vi "Add Scalar to Group.vi"(8 "error in":errorcluster, 10 "Scalar Data":T5, 11 "FPGA Addon refnum in":T2 format="%.0x") -> (0 "error out":errorcluster, 2 "Group Scalar Data out":T1 {"Scalar Section ref" format="%.0x"; "Group Section ref" format="%.0x"; "Group Scalar Registers"."Data Type" format="%.0x"}, 3 "FPGA Addon refnum out":T2=18446744073709551615 format="%.0x")   [LabVIEW 2019, in "Scripting API.lvlib"]
uses:
  Scripting API.lvlib
  TypeDefs/Input Scalar Data.ctl
  <vilib>/NI VeriStand/Custom Device API/Custom Device Item Ref.ctl
  TypeDefs/Group Scalar Data.ctl
  Addon/Addon Shared/Types/Register Information.ctl
  Addon/Addon Shared/Types/FPGA Addon Data Type.ctl
  Addon/Addon System Explorer/FPGA Addon System Explorer.lvlib
  Addon/Addon Shared/FPGA Addon Shared.lvlib
  <vilib>/NI VeriStand/Custom Device API/Custom Device API.lvlib
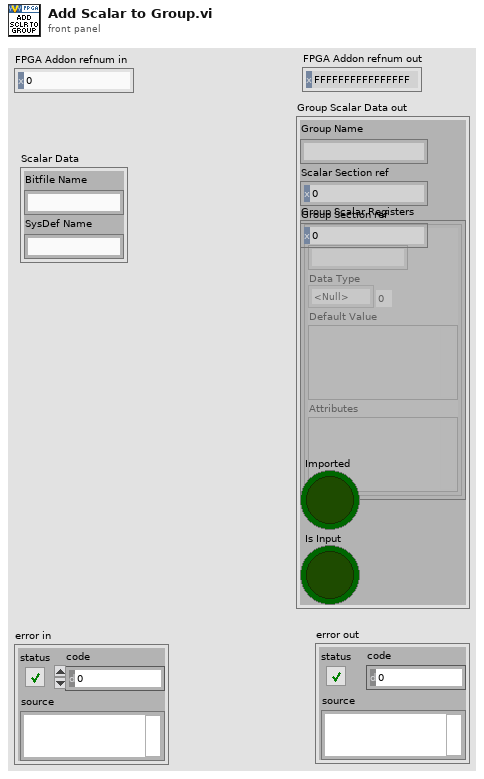
[diagram p1: front panel]
types:
  T1 = typedef "Scripting API.lvlib/Group Scalar Data.ctl" = cluster{"Group Name":string, "Scalar Section ref":T2, "Group Section ref":T2, "Group Scalar Registers":T3[], "Imported":bool, "Is Input":bool}
  T2 = typedef "Custom Device API.lvlib/Custom Device Item Ref.ctl" = u64
  T3 = typedef "FPGA Addon Shared.lvlib/Register Information.ctl" = cluster{"Name":string, "Data Type":T4, "Default Value":variant, "Attributes":variant}
  T4 = typedef "FPGA Addon Shared.lvlib/FPGA Addon Data Type.ctl" = enum8{"<Null>", "I8", "I16", "I32", "I64", "U8", "U16", "U32", "U64", "SGL", "Boolean", "Analog PWM In Settings", "Analog PWM In", "Digital PWM In Settings", "Digital PWM In", "Digital PWM Out", "Sine Out", "FXP", "FXP+/-24.5", "FXP+/-16.5", "FXP+/-32.8", "FXP+/-64.32", "FXP+/-16.7", "FXP+/-20.5", "FXP+/-27.5", "FXP+/-32.16", "FXP+16.3", "FXP+18.3", "Digital Static In", "Digital Static Out", "Digital Static In Settings", "Digital WSS Out", "Quad Encoder Settings", "Quad Encoder In", "Group"}
  T5 = typedef "Scripting API.lvlib/Input Scalar Data.ctl" = cluster{"Bitfile Name":string, "SysDef Name":string}
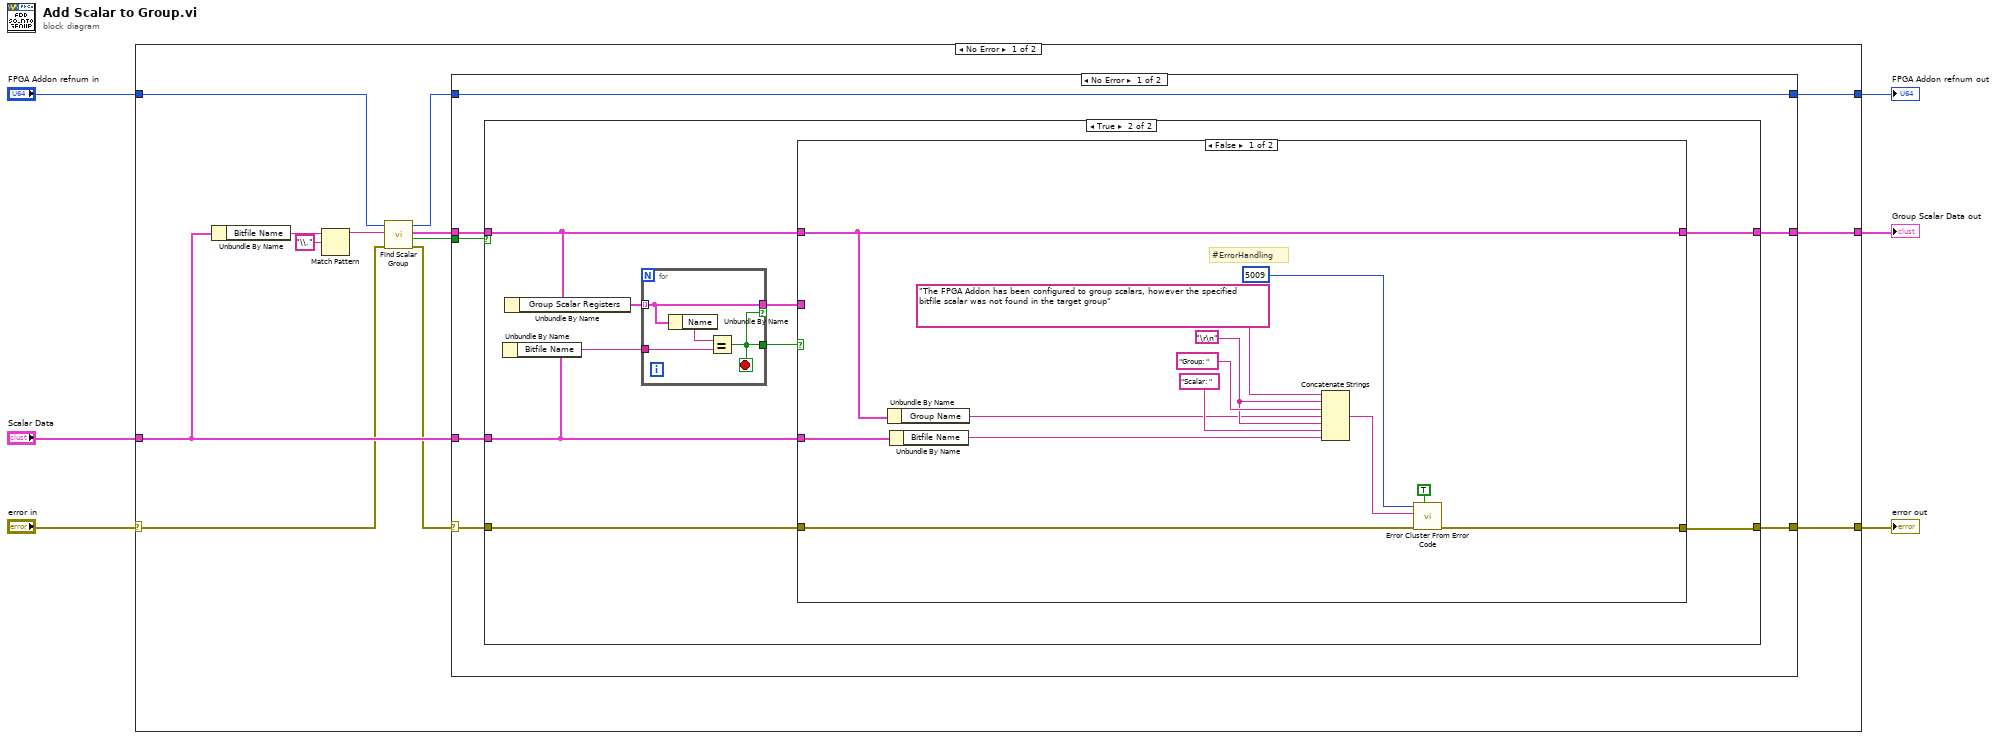
[diagram p0: block diagram]
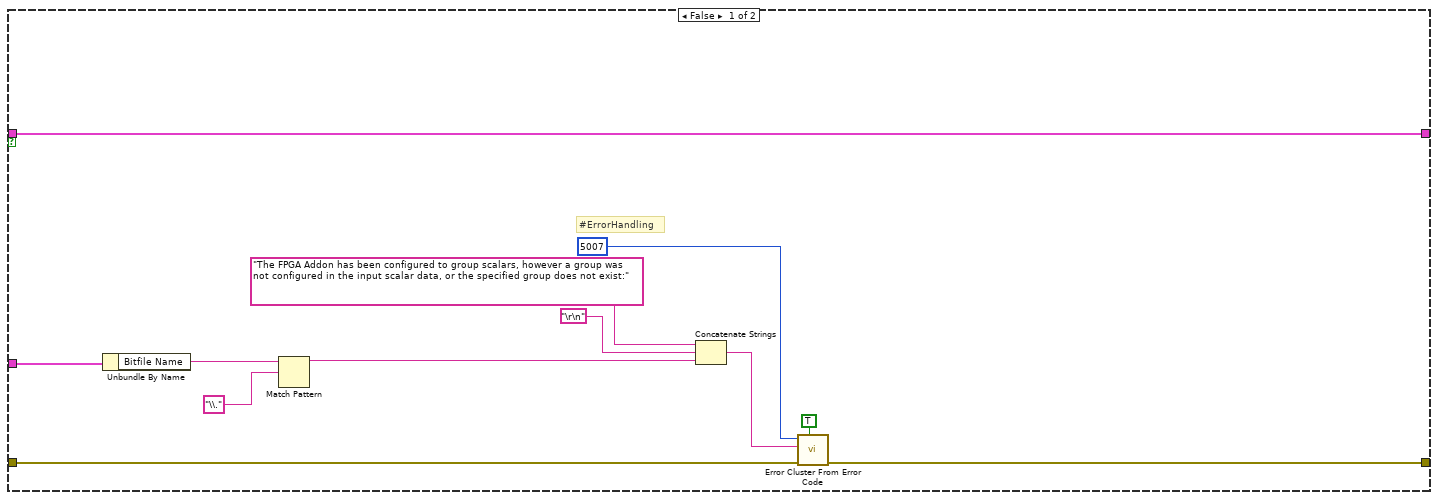
[diagram p2: hidden frame]
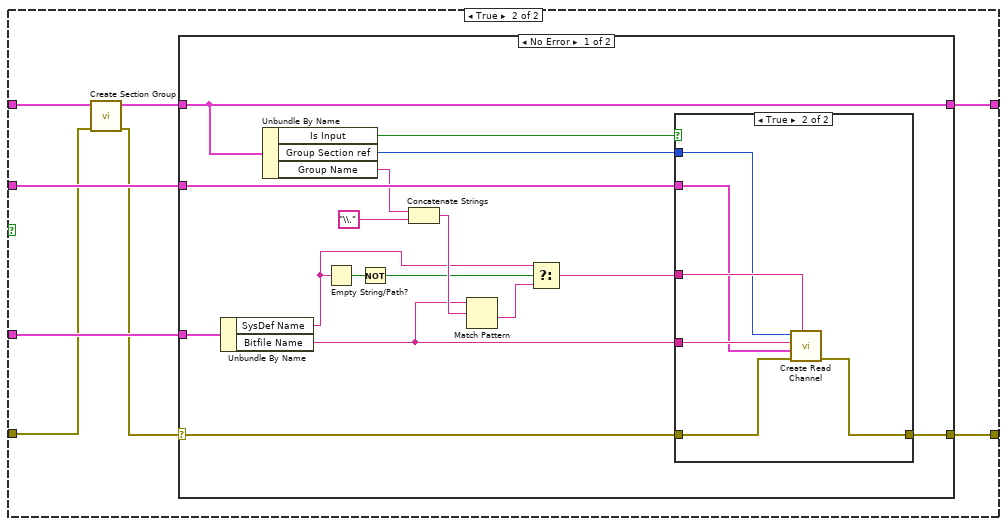
[diagram p3: hidden frame]
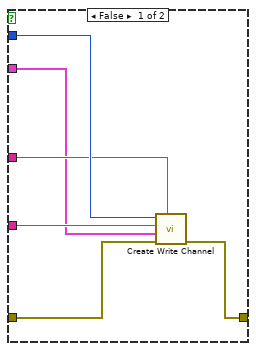
[diagram p4: hidden frame]
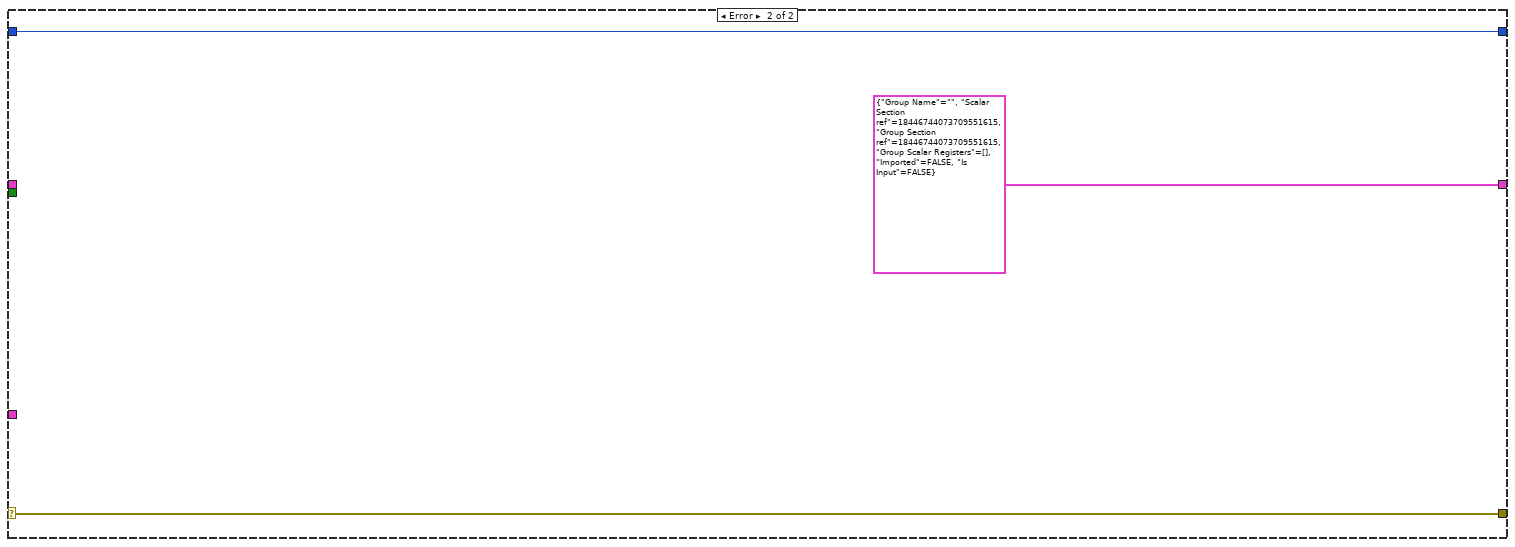
[diagram p6: hidden frame]
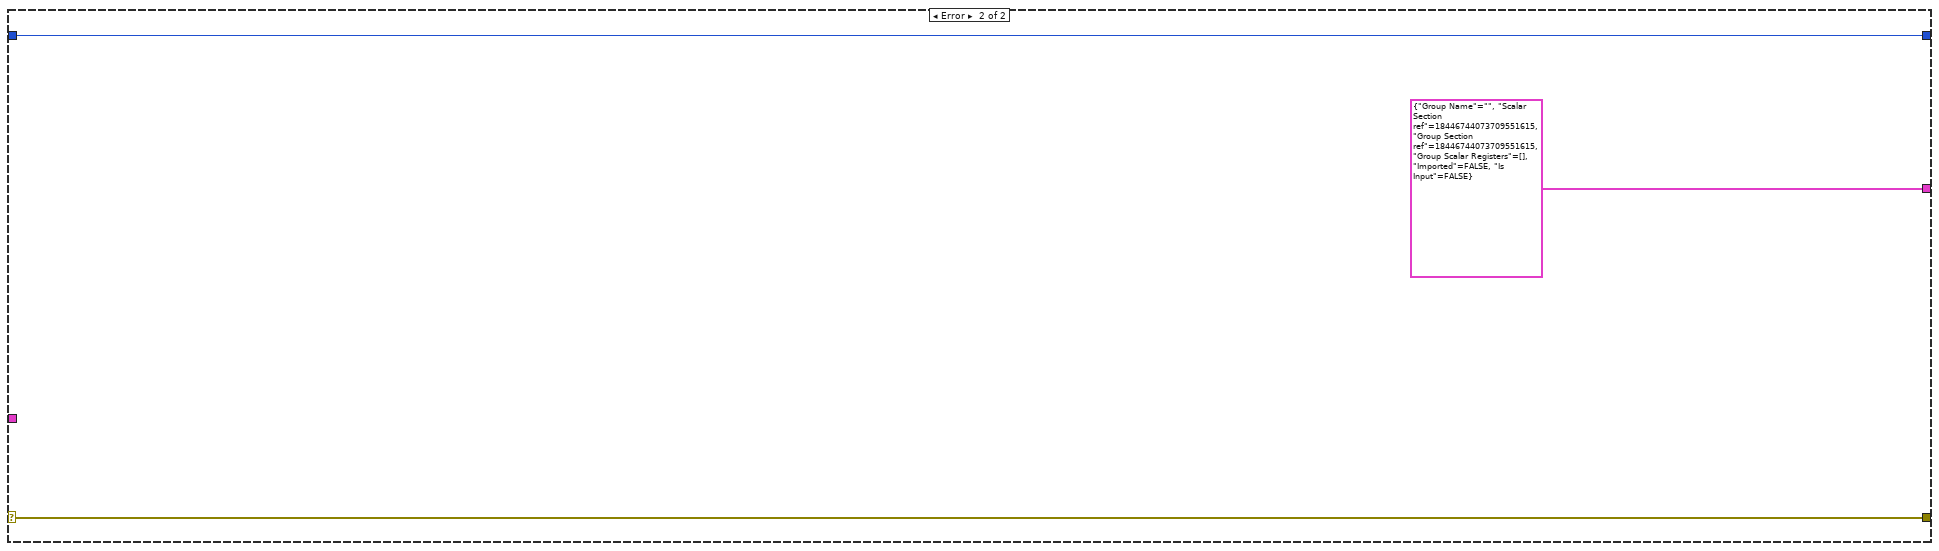
[diagram p7: hidden frame]
diagram:
  n1 = case shown="No Error" "error in" {
    selector: "error in" -> [w12 w108]
    tunnel: "Scalar Data" -> [w19 _]
    tunnel: "FPGA Addon refnum in" -> [w15 w107]
    tunnel: [w11 w108] -> w3
    tunnel: [w8 w107] -> w2
    tunnel: [w7 T1 {"Group Name"="", "Scalar Section ref"=18446744073709551615, "Group Section ref"=18446744073709551615, "Group Scalar Registers"=[], "Imported"=FALSE, "Is Input"=FALSE}] -> w1
    frame No Error {
      n2 = Unbundle By Name(w19) -> ("Bitfile Name"=w18:string)
      n3 = Match Pattern(string=w18, regular expression="\\.") -> (before substring=w14:string)  [unwired: 1 in, 3 out]
      n4 = call "Find Scalar Group.vi"("error in"=w12, "Group Name"=w14, "FPGA Addon refnum in"=w15) -> ("error out"=w10:errorcluster, "Found ?"=w16:bool, "Group Scalar Data"=w17:T1, "FPGA Addon refnum out"=w9:T2)  [unwired: 5 in]
      n5 = case shown="No Error" w10 {
        selector: w10 -> [w22 w105]
        tunnel: w19 -> [w26 _]
        tunnel: w17 -> [w25 _]
        tunnel: w16 -> [w24 _]
        tunnel: [w23 w105] -> w11
        tunnel: w9 -> [w21 w104]
        tunnel: [w21 w104] -> w8
        tunnel: [w20 T1 {"Group Name"="", "Scalar Section ref"=18446744073709551615, "Group Section ref"=18446744073709551615, "Group Scalar Registers"=[], "Imported"=FALSE, "Is Input"=FALSE}] -> w7
        frame No Error {
          n6 = case shown="True" w24 {
            tunnel: w25 -> [w38 w45]
            tunnel: w26 -> [w33 w42]
            tunnel: w22 -> [w35 w41]
            tunnel: [w34 w40] -> w23
            tunnel: [w38 w39] -> w20
            frame False {
              # "#ErrorHandling"
              n7 = Unbundle By Name(w33) -> ("Bitfile Name"=w31:string)
              n8 = Match Pattern(string=w31, regular expression="\\.") -> (before substring=w30:string)  [unwired: 1 in, 3 out]
              n9 = Concatenate Strings("The FPGA Addon has been configured to group scalars, however a group was not configured in the input scalar data, or the specified group does not exist:" ("error message (\"\")"), "\r\n", w30) -> (w27:string)
              n10 = call <vilib>:"Error Cluster From Error Code.vi"("show call chain? (False)"=TRUE, "error in (no error)"=w35, "error message (\"\")"=w27, "error code (0)"=5007) -> ("error out"=w34:errorcluster)  [unwired: 5 in]
            }
            frame True {
              n11 = Unbundle By Name(w42) -> ("Bitfile Name"=w43:string)
              n12 = Unbundle By Name(w45) -> ("Group Scalar Registers"=w47:T3[])
              n13 = for {
                tunnel: w47 -> [w100] mode=indexing
                tunnel: w43 -> [w101]
                tunnel: [w100] -> w44 if=w99
                tunnel: [w99] -> w46
                stop <- w99 stop-if-true
                n14 = Unbundle By Name(w100) -> ("Name"=w102:string)
                n15 = Equal?(x=w102, y=w101) -> (x = y?=w99:bool)
              }
              n16 = case shown="False" w46 {
                tunnel: w45 -> [w49 w68]
                tunnel: w44 -> [_ w66]
                tunnel: w42 -> [w51 w67]
                tunnel: w41 -> [w56 w65]
                tunnel: [w55 w63] -> w40
                tunnel: [w49 w61] -> w39
                frame False {
                  w53 = "\r\n"
                  # "#ErrorHandling"
                  n17 = Unbundle By Name(w49) -> ("Group Name"=w48:string)
                  n18 = Unbundle By Name(w51) -> ("Bitfile Name"=w50:string)
                  n19 = Concatenate Strings("The FPGA Addon has been configured to group scalars, however the specified bitfile scalar was not found in the target group" ("error message (\"\")"), w53, "Group: " ("string"), w48, w53, "Scalar: " ("string"), w50) -> (w57:string)
                  n20 = call <vilib>:"Error Cluster From Error Code.vi"("show call chain? (False)"=TRUE, "error in (no error)"=w56, "error message (\"\")"=w57, "error code (0)"=5009) -> ("error out"=w55:errorcluster)  [unwired: 5 in]
                }
                frame True {
                  n21 = call "Create Section Group.vi"("error in"=w65, "Group Scalar Data in"=w68) -> ("error out"=w64:errorcluster, "Group Scalar Data out"=w62:T1)  [unwired: 8 in]
                  n22 = case shown="No Error" w64 {
                    selector: w64 -> [w71 w98]
                    tunnel: w67 -> [w84 _]
                    tunnel: w66 -> [w73 _]
                    tunnel: [w70 w98] -> w63
                    tunnel: w62 -> [w69 w97]
                    tunnel: [w69 w97] -> w61
                    frame No Error {
                      n23 = Unbundle By Name(w84) -> ("SysDef Name"=w79:string, "Bitfile Name"=w74:string)
                      n24 = Unbundle By Name(w69) -> ("Is Input"=w76:bool, "Group Section ref"=w75:T2, "Group Name"=w72:string)
                      n25 = Empty String/Path?(string/path=w79) -> (empty?=w81:bool)
                      n26 = Not(x=w81) -> (.not. x?=w80:bool)
                      n27 = Concatenate Strings(w72, "\\.") -> (w82:string)
                      n28 = Match Pattern(string=w74, regular expression=w82) -> (after substring=w78:string)  [unwired: 1 in, 3 out]
                      n29 = Select(t=w79, s=w80, f=w78) -> (s? t:f=w77:string)
                      n30 = case shown="True" w76 {
                        tunnel: w77 -> [w89 w96]
                        tunnel: w75 -> [w90 w95]
                        tunnel: w74 -> [w88 w94]
                        tunnel: w73 -> [w87 w93]
                        tunnel: w71 -> [w86 w92]
                        tunnel: [w85 w91] -> w70
                        frame False {
                          n31 = call "Create Write Channel.vi"("Name"=w89, "error in (no error)"=w86, "Cluster"=w87, "Bitfile Name"=w88, "Item Ref in"=w90) -> ("error out"=w85:errorcluster)  [unwired: 6 in]
                        }
                        frame True {
                          n32 = call "Create Read Channel.vi"("Name"=w96, "error in (no error)"=w92, "Channel"=w93, "Bitfile Name"=w94, "Item Ref in"=w95) -> ("error out"=w91:errorcluster)  [unwired: 6 in]
                        }
                      }
                    }
                    frame Error {
                    }
                  }
                }
              }
            }
          }
        }
        frame Error {
        }
      }
    }
    frame Error {
    }
  }
  "error out" <- w3
  "FPGA Addon refnum out" <- w2
  "Group Scalar Data out" <- w1
